vi "GetThirdAxis.vi"(2 "1st Axis":u16, 3 "2nd Axis":u16) -> (0 "3rd Axis":i32)   [LabVIEW 2009]
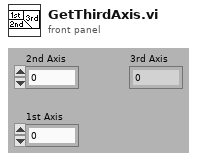
[diagram p1: front panel]
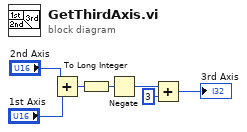
[diagram p0: block diagram]
diagram:
  n1 = Add(x="2nd Axis", y="1st Axis") -> (x+y=w1:u16)
  n2 = To Long Integer(number=w1) -> (32bit integer=w2:i32)
  n3 = Negate(x=w2) -> (-x=w3:i32)
  n4 = Add(x=w3, y=3) -> (x+y=→"3rd Axis":i32)
